vi "Read Current (Logarithmic Voltage Sweep).vi"(5 "Delay Time (0.01 S)":dbl=0.01, 6 "Pulse Stop Level (10 V)":dbl=10.0, 7 "Sweep Points (5)":i32=5, 8 "error in (no error)":errorcluster, 9 "Pulse Start Level (1 V)":dbl=1.0, 10 "Source Measure Unit Channel (0: Channel A)":i32(ring) items=["Channel A", "Channel B"], 11 "VISA resource name":refnum<visa-resource-name>) -> (0 "error out":errorcluster, 2 "Current (A)":dbl[](array[numeric]), 3 "VISA resource name out":refnum<visa-resource-name>)   [LabVIEW 2017, in "Keithley 2600 Series.lvlib"]
doc: "Performs a logarithmic voltage sweep with current measured at every point."
uses:
  <instrlib>/Keithley 2600 Series/Keithley 2600 Series.lvlib
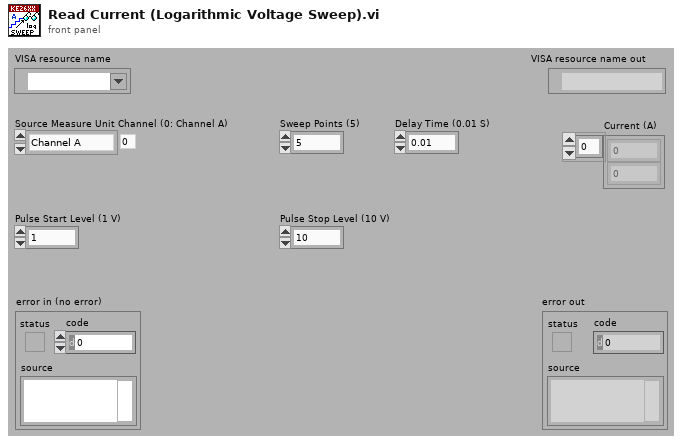
[diagram p1: front panel]
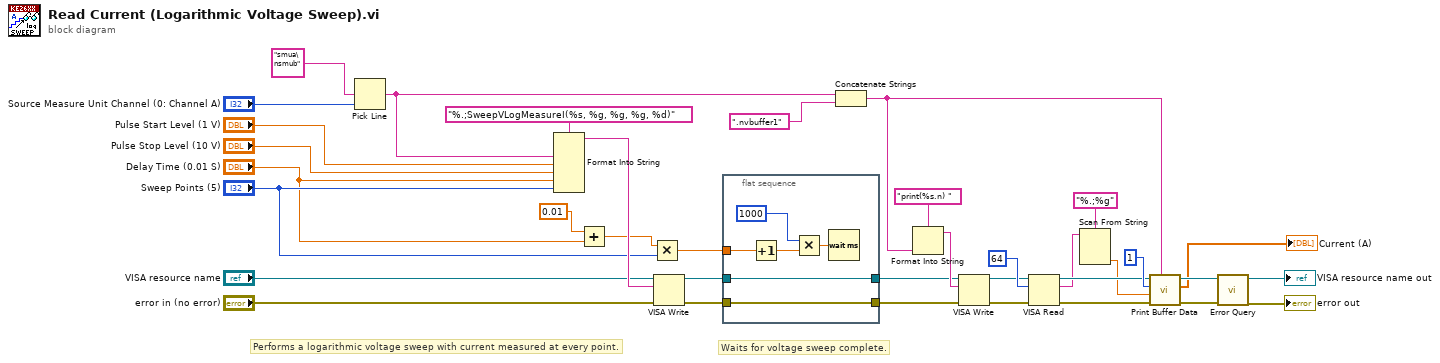
[diagram p0: block diagram]
diagram:
  # "Waits for voltage sweep complete."
  # "Performs a logarithmic voltage sweep with current measured at every point."
  n1 = Pick Line(multi-line string="smua\nsmub", line index="Source Measure Unit Channel (0: Channel A)") -> (output string=w6:string)  [unwired: 1 in]
  n2 = Format Into String(format string="%.;SweepVLogMeasureI(%s, %g, %g, %g, %d)", w6, "Pulse Start Level (1 V)", "Pulse Stop Level (10 V)", "Delay Time (0.01 S)", "Sweep Points (5)") -> (resulting string=w33:string)  [unwired: 2 in, 1 out]
  n3 = Add(x=0.01, y="Delay Time (0.01 S)") -> (x+y=w21:dbl)
  n4 = Multiply(x=w21, y="Sweep Points (5)") -> (x*y=w20:dbl)
  n5 = VISA Write(VISA resource name="VISA resource name", write buffer=w33, error in (no error)="error in (no error)") -> (VISA resource name out=w26:refnum<visa-resource-name>, error out=w25:errorcluster)  [unwired: 1 out]
  n6 = flat-sequence {
    tunnel: w26 -> [w42]
    tunnel: w25 -> [w41]
    tunnel: [w42] -> w5
    tunnel: [w41] -> w4
    tunnel: w20 -> [w40]
    frame #0 {
      n7 = Increment(x=w40) -> (x+1=w39:dbl)
      n8 = Multiply(x=1000, y=w39) -> (x*y=w37:dbl)
      n9 = Wait (ms)(milliseconds to wait=w37) -> ()  [unwired: 1 out]
    }
  }
  n10 = Concatenate Strings(w6, ".nvbuffer1" ("string")) -> (w7:string)
  n11 = Format Into String(format string="print(%s.n) ", w7) -> (resulting string=w9:string)  [unwired: 2 in, 1 out]
  n12 = VISA Write(VISA resource name=w5, write buffer=w9, error in (no error)=w4) -> (VISA resource name out=w12:refnum<visa-resource-name>, error out=w11:errorcluster)  [unwired: 1 out]
  n13 = VISA Read(VISA resource name=w12, byte count=u32 64, error in (no error)=w11) -> (VISA resource name out=w17:refnum<visa-resource-name>, read buffer=w15:string, error out=w16:errorcluster)  [unwired: 1 out]
  n14 = Scan From String(format string="%.;%g", input string=w15) -> (output 1=w14:dbl)  [unwired: 3 in, 3 out]
  n15 = call <instrlib>:"Print Buffer Data.vi"("Reading Buffer (smua.nvbuffer1)"=w7, "error in (no error)"=w16, "End Index (1)"=w14, "Start Index (1)"=1 ("Start Index (0)"), "VISA resource name"=w17) -> ("error out"=w2:errorcluster, "Buffer Data"=→"Current (A)":dbl[], "VISA resource name out"=w3:refnum<visa-resource-name>)  [unwired: 4 in]
  n16 = call <instrlib>:"Error Query.vi"("error in (no error)"=w2, "VISA resource name"=w3) -> ("error out"=→"error out":errorcluster, "VISA resource name out"=→"VISA resource name out":refnum<visa-resource-name>)  [unwired: 6 in, 2 out]
